vi "2 wind_degree_shift.vi"(1 "Wind Theta -180 - 180":dbl) -> (0 "Wind Theta 0-360":dbl)   [LabVIEW 2011]
doc: "Changes wind range from [-180:180] to [0:360]"
panel:
  # "Convert equivalent angles from negative to positive"
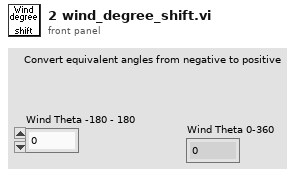
[diagram p1: front panel]
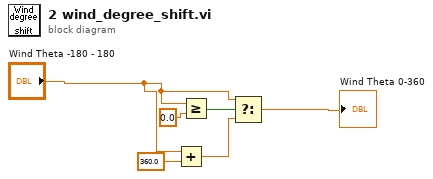
[diagram p0: block diagram]
diagram:
  n1 = Add(x="Wind Theta -180 - 180", y=360.0) -> (x+y=w3:dbl)
  n2 = Greater Or Equal?(x="Wind Theta -180 - 180", y=0.0) -> (x >= y?=w5:bool)
  n3 = Select(t="Wind Theta -180 - 180", s=w5, f=w3) -> (s? t:f=→"Wind Theta 0-360":dbl)
